vi "Shooter Controller Initialization.vi"(10 "Subsystem Name":string, 11 "Default Command":T1) -> (3 "Current Command":T6)   [LabVIEW 2020]
doc: "This VI is called once for the subsystem. It allocates the notifier and combines the timing, default command, and other information into a single data wire."
uses:
  Shooter Setpoints.ctl
  Shooter Operations.ctl
  <vilib>/Rock Robotics/WPI/Framework/Command Status Info.ctl
  <vilib>/Rock Robotics/WPI/Framework/Completion Status.ctl
  <vilib>/Rock Robotics/WPI/Framework/Completion Notifier.ctl
  Shooter Published Globals.vi
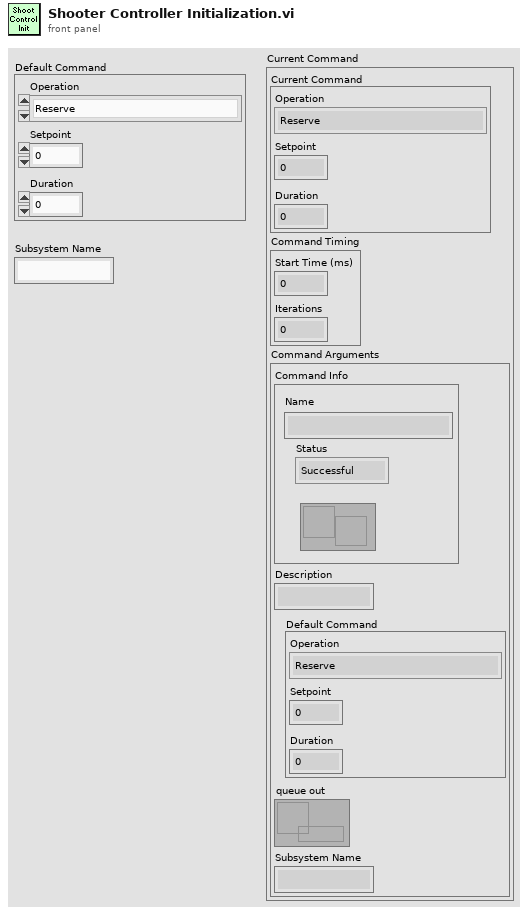
[diagram p1: front panel]
types:
  T1 = typedef "Shooter Setpoints.ctl" = cluster{"Operation":T2, "Setpoint":dbl, "Duration":dbl}
  T2 = typedef "Shooter Operations.ctl" = enum16{"Reserve", "Read Current", "Immediate", "For Time ", "Stop"}
  T3 = typedef "Command Status Info.ctl" = cluster{"Name":string, "Status":T4, "notifier out":T5}
  T4 = typedef "Completion Status.ctl" = enum16{"Successful", "Aborted", "Incomplete"}
  T5 = typedef "Completion Notifier.ctl" = refnum<notifier>
  T6 = cluster{"Current Command":T1, "Command Timing":cluster{"Start Time (ms)":u32, "Iterations":i32}, "Command Arguments":cluster{"Command Info":T3, "Description":string, "Default Command":T1, "queue out":refnum<queue>, "Subsystem Name":string}}
  T7 = cluster{"Default Command":T1, "Command Info":T3, "Description":string}
  T8 = cluster{"Command Info":T3, "Description":string, "Default Command":T1, "queue out":refnum<queue>, "Subsystem Name":string}
  T9 = cluster{"Default Command":T1, cluster{"Start Time (ms)":u32, "Iterations":i32}, cluster{"Command Info":T3, "Description":string, "Default Command":T1, "queue out":refnum<queue>, "Subsystem Name":string}}
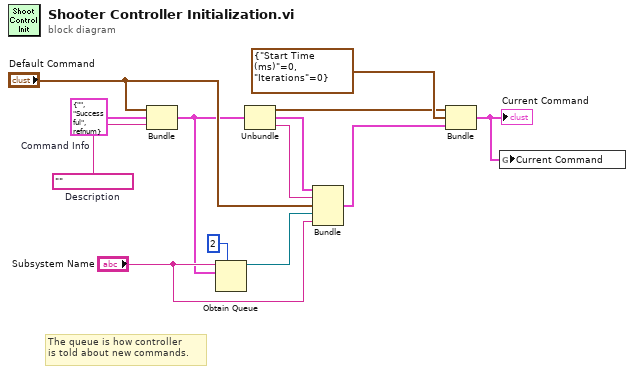
[diagram p0: block diagram]
diagram:
  w10 = T3 {"Name"="", "Status"=enum."Successful", "notifier out"=refnum}  # Command Info
  w11 = ""  # Description
  # "The queue is how controller\nis told about new commands."
  n1 = Bundle("Default Command"="Default Command", "Command Info"=w10, "Description"=w11) -> (w4:T7)  [unwired: 1 in]
  n2 = Obtain Queue(max queue size (-1, unlimited)=2, name (unnamed)="Subsystem Name", element data type=w4) -> (queue out=w3:refnum<queue>)  [unwired: 2 in, 2 out]
  n3 = Unbundle(w4) -> ("Default Command"=w12:T1, "Command Info"=w7:T3, "Description"=w8:string)
  n4 = Bundle("Command Info"=w7, "Description"=w8, "Default Command"="Default Command", "queue out"=w3, "Subsystem Name"="Subsystem Name") -> (w9:T8)  [unwired: 1 in]
  n5 = Bundle("Default Command"=w12, cluster{"Start Time (ms)":u32, "Iterations":i32} {"Start Time (ms)"=0, "Iterations"=0}, w9) -> (w1:T9)  [unwired: 1 in]
  "Current Command" <- w1
  n6 = global write "Shooter Published Globals.vi" "Current Command"(w1) -> ()
